vi "Main.vi"() -> ()   [LabVIEW 2017]
uses:
  <vilib>/Utility/file.llb/Read Delimited Spreadsheet (string).vi
  <vilib>/Utility/file.llb/Write Delimited Spreadsheet (string).vi
panel:
  in  "Done":bool
  in  "configuration file path":path
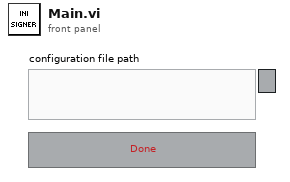
[diagram p1: front panel]
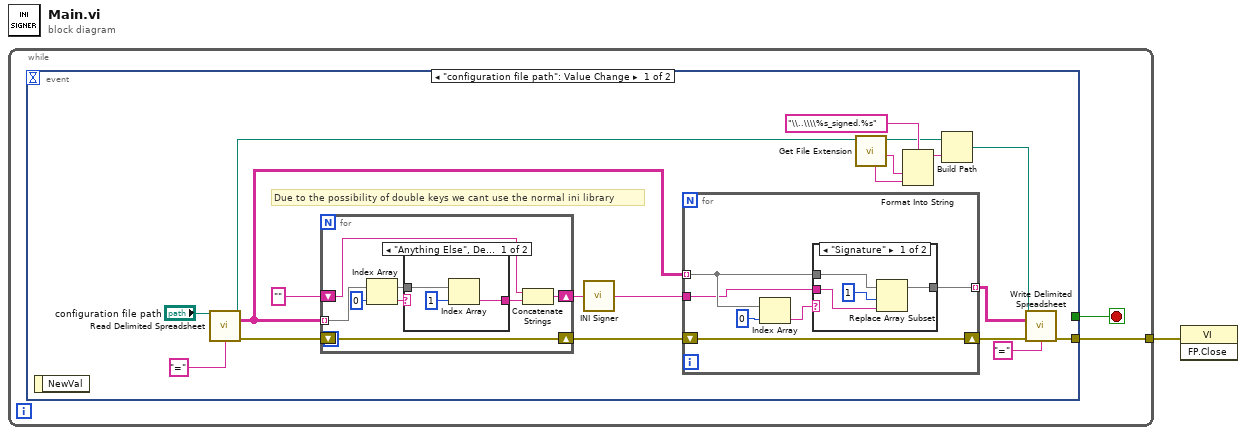
[diagram p0: block diagram]
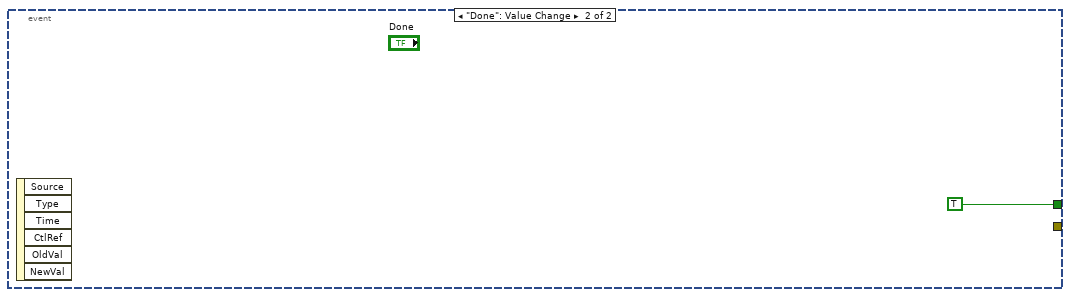
[diagram p4: hidden frame]
diagram:
  n1 = while {
    tunnel: [w2] -> w1
    stop <- w3 stop-if-true
    n2 = event shown="[0] \"configuration file path\": Value Change" {
      selector: _ -> [_ _]
      dyn-events: _ -> [_ _]
      timeout: _ -> [_ _]
      tunnel: [_ TRUE] -> w3
      tunnel: [w11 _] -> w2
      event "configuration file path": Value Change {
        # "Due to the possibility of double keys we cant use the normal ini library"
        n3 = event-data() -> ()  [unwired: 1 in, 1 out]
        n4 = call-poly <vilib>:"Read Delimited Spreadsheet.vi"("file path (dialog if empty)"="configuration file path", "delimiter (\\t)"="=" ("delimiter (\\t)")) -> ("new file path (Not A Path if cancelled)"=w10:path, "all rows"=w17:string[][], "error out"=w20:errorcluster)  [unwired: 8 in, 3 out]
        n5 = for {
          tunnel: w17 -> [w37] mode=indexing
          shift-right: [w35] -> w16
          shift-left: w20 -> [w35]
          shift-right: [w39] -> w18
          shift-left: "" -> [w38]
          n6 = Index Array(array=w37, index=0) -> (element=w34:string)
          n7 = case shown="\"Anything Else\", Default" w34 {
            tunnel: w37 -> [w42 _]
            tunnel: [w41 _] -> w36
            frame "Anything Else", Default {
              n8 = Index Array(array=w42, index=1) -> (element=w41:string)
            }
            frame "IsPrimary", "Signature" {
            }
          }
          n9 = Concatenate Strings(w38, w36) -> (w39:string)
        }
        n10 = call "INI Signer.vi"("String Key Values"=w18) -> ("Signature"=w14:string)
        n11 = for {
          tunnel: w17 -> [w27] mode=indexing
          shift-right: [w26] -> w13
          shift-left: w16 -> [w26]
          tunnel: w14 -> [w24]
          tunnel: [w23] -> w12 mode=indexing
          n12 = Index Array(array=w27, index=0) -> (element=w25:string)
          n13 = case shown="\"Signature\"" w25 {
            tunnel: w27 -> [w32 w33]
            tunnel: w24 -> [w30 _]
            tunnel: [w29 w33] -> w23
            frame "Signature" {
              n14 = Replace Array Subset(array=w32, new element=w30, index=1) -> (w29:string[])
            }
            frame "Anything else", Default {
            }
          }
        }
        n15 = call <vilib>:"Get File Extension.vi"("file"=w10) -> ("filename without extension"=w9:string, "dup file"=w6:path, "unmodified file extension"=w8:string)  [unwired: 6 in, 2 out]
        n16 = Format Into String(format string="\\..\\\\%s_signed.%s", w9, w8) -> (resulting string=w5:string)  [unwired: 2 in, 1 out]
        n17 = Build Path(base path=w6, name or relative path=w5) -> (appended path=w4:path)
        n18 = call-poly <vilib>:"Write Delimited Spreadsheet.vi"("file path (dialog if empty)"=w4, "2D data"=w12, "error in (no error)"=w13, "delimiter (\\t)"="=" ("delimiter (\\t)")) -> ("error out"=w11:errorcluster)  [unwired: 10 in, 1 out]
      }
      event "Done": Value Change {
        n19 = event-data() -> ()  [unwired: 1 in, 6 out]
      }
    }
  }
  n20 = invoke class="VI" method="FP.Close"(error in=w1) -> ()  [unwired: 2 in, 3 out]
